vi "AI@ClassifyEditor__Parameter.vi"(1 "ParamterIn":string) -> (0 "ParamterOut":string)   [LabVIEW 2020]
uses:
  MainFrame/Global.vi
  <vilib>/vision/NI_Vision_Development_Module.lvlib
panel:
  out "Image":T1(plugin-control)
  in  "Preview":bool
  in  "SubDir":string(combo)
  in  "Capture":string(combo)
  in  "Confirm":bool
  # "AI@ClassifyEditor $Capture(\\$Directory)"
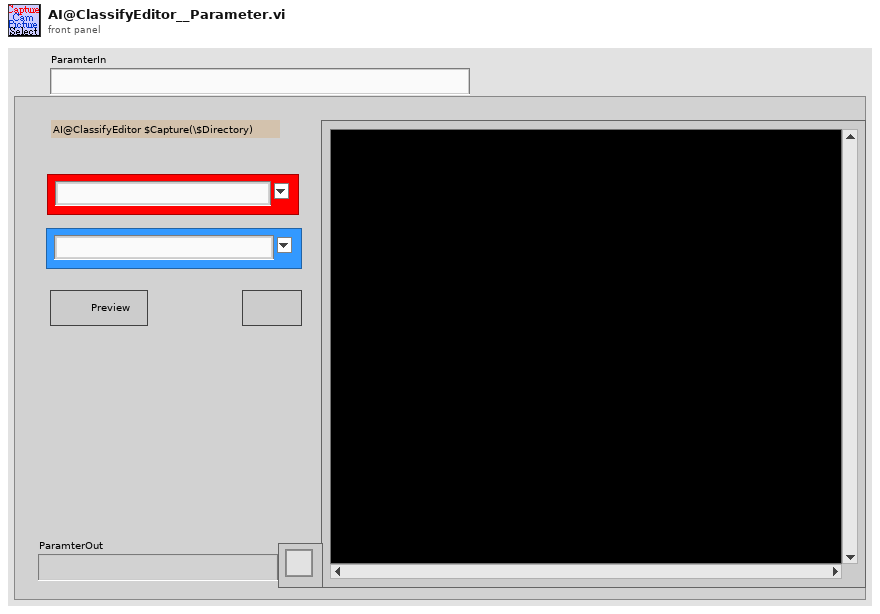
[diagram p1: front panel]
types:
  T1 = typedef "IMAQ Image.ctl" = refnum<image>
  T2 = cluster{"Browser Size":cluster{"X":i32, "Y":i32}, "Images per Line":i32, "Background Color":u32, "Frame Size":i32, "Frame Style":u16}
  T3 = typedef "Image Type" = u32
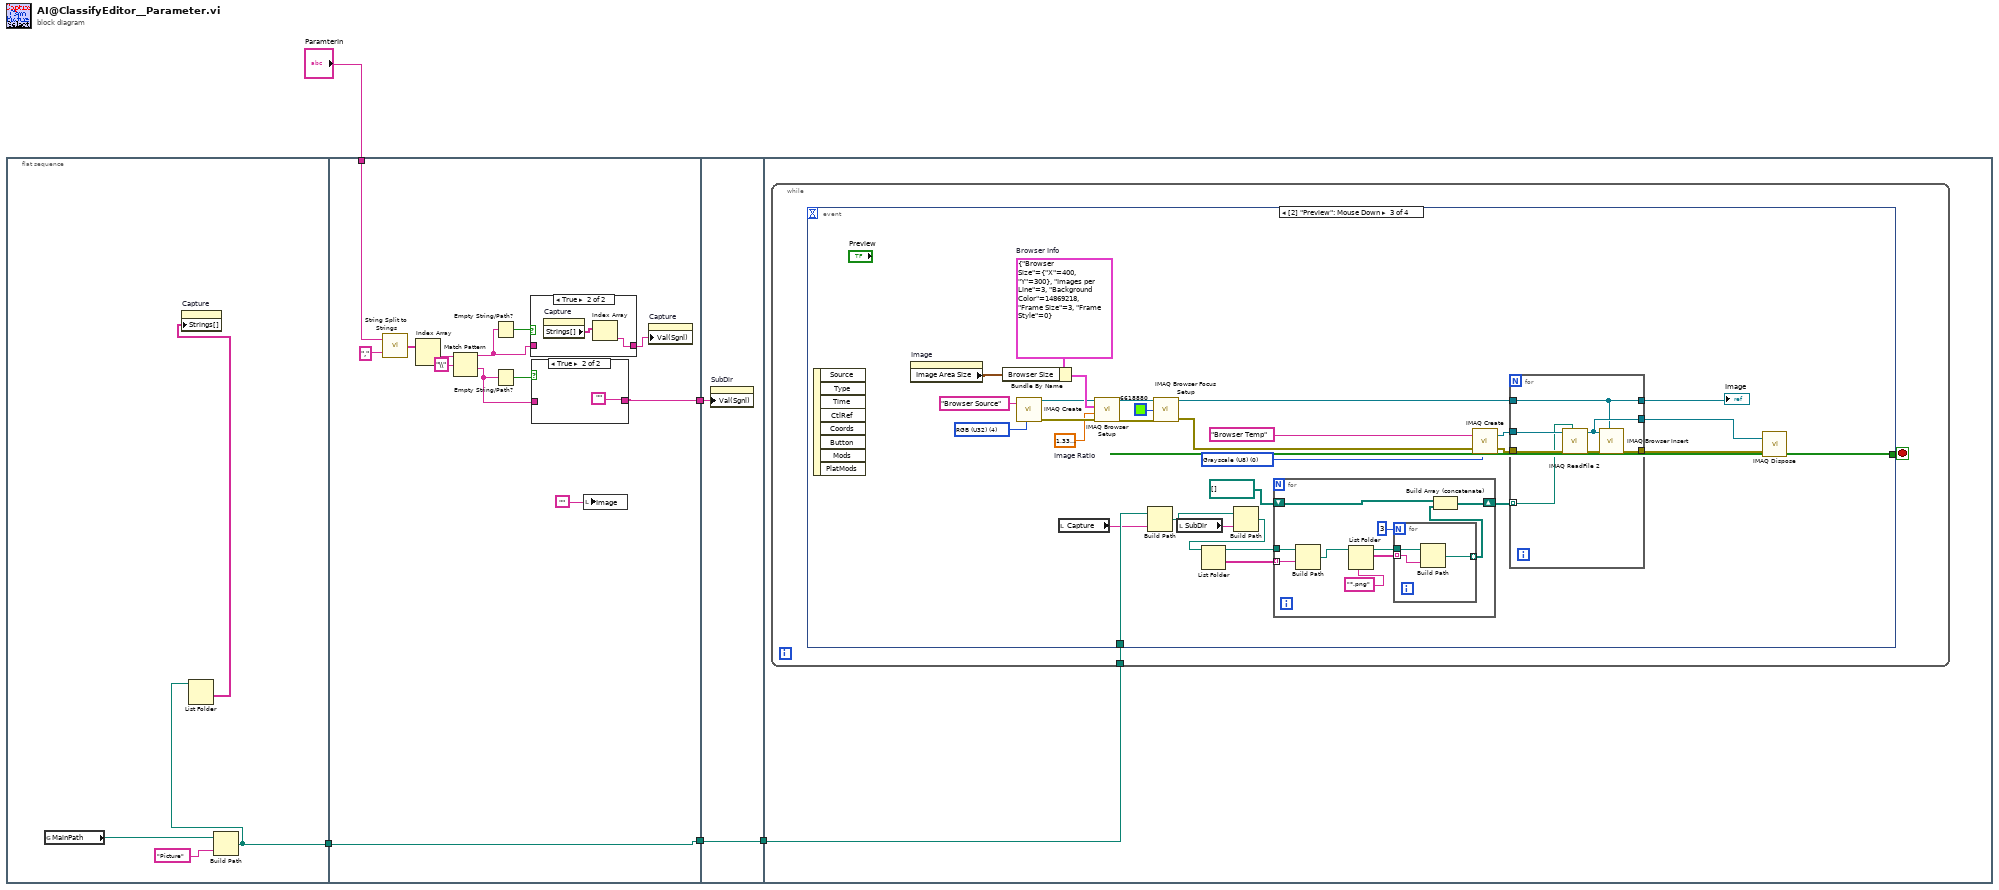
[diagram p0: block diagram]
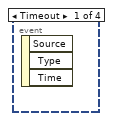
[diagram p4: hidden frame]
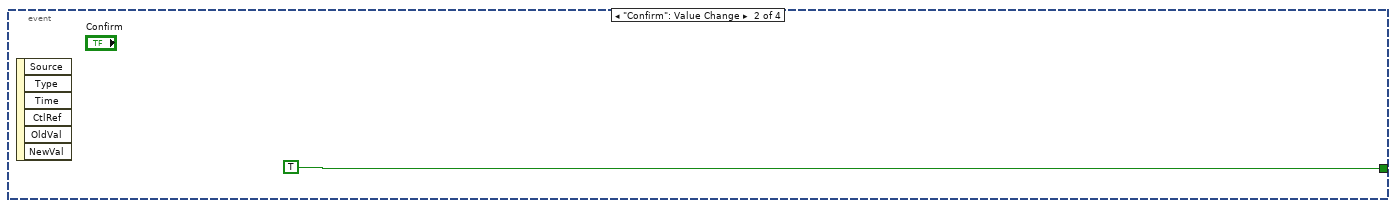
[diagram p5: hidden frame]
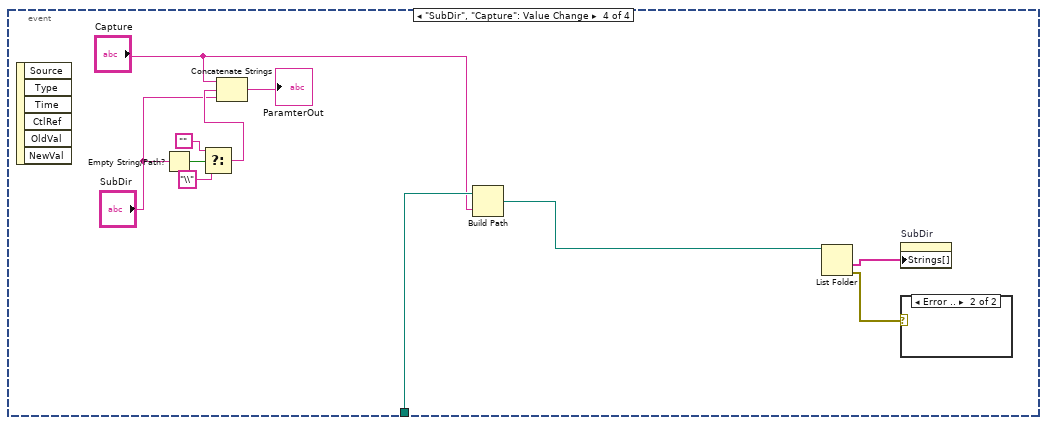
[diagram p6: hidden frame]
diagram:
  n1 = flat-sequence {
    tunnel: [w7] -> w2
    tunnel: "ParamterIn" -> [w20]
    tunnel: [w18] -> w3
    tunnel: w2 -> [w18]
    tunnel: [w17] -> w1
    tunnel: [w29] -> w4
    tunnel: w3 -> [w29]
    tunnel: w1 -> [w28]
    tunnel: w4 -> [w30]
    frame #0 {
      n2 = global read "Global.vi" "MainPath"() -> (w8:path)
      n3 = Build Path(base path=w8, name or relative path="Picture") -> (appended path=w7:path)
      n4 = List Folder(path=w7) -> (folder names=w6:string[])  [unwired: 3 in, 3 out]
      n5 = property on="Capture" class="CmbBox"("Strings[]"=w6) -> ()  [unwired: 2 in, 2 out]
    }
    frame #1 {
      n6 = call "String Split to Strings.vi"("search string/char (-)"=",", "String"=w20) -> ("Array"=w22:string[])
      n7 = Index Array(array=w22) -> (element #1=w14:string)  [unwired: 2 in, 1 out]
      n8 = Match Pattern(string=w14, regular expression="\\") -> (before substring=w12:string, after substring=w11:string)  [unwired: 1 in, 2 out]
      n9 = Empty String/Path?(string/path=w12) -> (empty?=w19:bool)
      n10 = Empty String/Path?(string/path=w11) -> (empty?=w15:bool)
      n11 = case shown="True" w19 {
        tunnel: w12 -> [w25 _]
        tunnel: [w25 w26] -> w16
        frame False {
        }
        frame True {
          n12 = property on="Capture" class="CmbBox"() -> ("Strings[]"=w27:string[])  [unwired: 2 in, 2 out]
          n13 = Index Array(array=w27) -> (element=w26:string)  [unwired: 1 in]
        }
      }
      n14 = case shown="True" w15 {
        tunnel: [w23 ""] -> w17
        tunnel: w11 -> [w23 _]
        frame False {
        }
        frame True {
        }
      }
      n15 = local write "Image"("") -> ()
      n16 = property on="Capture" class="CmbBox"("Val(Sgnl)"=w16) -> ()  [unwired: 2 in, 2 out]
    }
    frame #2 {
      n17 = property on="SubDir" class="CmbBox"("Val(Sgnl)"=w28) -> ()  [unwired: 2 in, 2 out]
    }
    frame #3 {
      n18 = while {
        tunnel: w30 -> [w31]
        stop <- w32 stop-if-true
        n19 = event shown="[2] \"Preview\": Mouse Down" {
          selector: _ -> [_ _ _ _]
          dyn-events: _ -> [_ _ _ _]
          timeout: _ -> [_ _ _ _]
          tunnel: [_ TRUE _ _] -> w32
          tunnel: w31 -> [_ _ w41 w91]
          event Timeout {
            n20 = event-data() -> ()  [unwired: 1 in, 3 out]
          }
          event "Confirm": Value Change {
            n21 = event-data() -> ()  [unwired: 1 in, 6 out]
          }
          event "Preview": Mouse Down {
            w43 = sgl 1.33  # Image Ratio
            w59 = T2 {"Browser Size"={"X"=400, "Y"=300}, "Images per Line"=3, "Background Color"=14869218, "Frame Size"=3, "Frame Style"=0}  # Browser Info
            w50 = T3 0 items=["Grayscale (U8)", "Grayscale (I16)", "Grayscale (SGL)", "Complex (CSG)", "RGB (U32)", "HSL (U32)", "RGB (U64)", "Grayscale (U16)"] ("Image Type")
            w48 = T3 4 items=["Grayscale (U8)", "Grayscale (I16)", "Grayscale (SGL)", "Complex (CSG)", "RGB (U32)", "HSL (U32)", "RGB (U64)", "Grayscale (U16)"] ("Image Type")
            n22 = event-data() -> ()  [unwired: 1 in, 8 out]
            n23 = property on="Image" class="ImageControl"() -> ("Image Area Size"=w60:cluster{"Width":u32, "Height":u32})  [unwired: 2 in, 2 out]
            n24 = Bundle By Name(cluster=w59, "Browser Size"=w60) -> (w61:T2)
            n25 = call "IMAQ Create"("Image Name"="Browser Source", "Image Type"=w48) -> ("New Image"=w46:T1, "error out"=w47:errorcluster)  [unwired: 3 in]
            n26 = local read "Capture"() -> (w40:string)
            n27 = call "IMAQ Browser Setup"("error in (no error)"=w47, "Image Ratio"=w43, "Browser Info"=w61, "Image In"=w46) -> ("error out"=w55:errorcluster, "Image Browser Out"=w54:T1)  [unwired: 2 out]
            n28 = Build Path(base path=w41, name or relative path=w40) -> (appended path=w39:path)
            n29 = call "IMAQ Browser Focus Setup"("error in (no error)"=w55, "Focus Color"=u32 6618880, "Image Browser In"=w54) -> ("error out"=w57:errorcluster, "Image Browser Out"=w56:T1)  [unwired: 1 in]
            n30 = local read "SubDir"() -> (w42:string)
            n31 = Build Path(base path=w39, name or relative path=w42) -> (appended path=w38:path)
            n32 = List Folder(path=w38) -> (path out=w37:path, folder names=w36:string[])  [unwired: 3 in, 2 out]
            n33 = for {
              tunnel: w37 -> [w65]
              tunnel: w36 -> [w64] mode=indexing
              shift-right: [w67] -> w34
              shift-left: path[] [] -> [w66]
              n34 = Build Path(base path=w65, name or relative path=w64) -> (appended path=w63:path)
              n35 = List Folder(path=w63, pattern="*.png") -> (path out=w70:path, filenames=w69:string[])  [unwired: 2 in, 2 out]
              n36 = for {
                N: 3 -> [_]
                tunnel: w70 -> [w75]
                tunnel: w69 -> [w74] mode=indexing
                tunnel: [w73] -> w68 mode=indexing
                n37 = Build Path(base path=w75, name or relative path=w74) -> (appended path=w73:path)
              }
              n38 = Build Array (concatenate)(w66, w68) -> (w67:path[])
            }
            n39 = call "IMAQ Create"("Image Name"="Browser Temp", "Image Type"=w50, "error in (no error)"=w57) -> ("New Image"=w52:T1, "error out"=w44:errorcluster)  [unwired: 2 in]
            n40 = for {
              tunnel: w56 -> [w77]
              tunnel: w44 -> [w81]
              tunnel: [w80] -> w45
              tunnel: [w77] -> w62
              tunnel: w52 -> [w79]
              tunnel: [w78] -> w53
              tunnel: w34 -> [w76] mode=indexing
              n41 = call "IMAQ ReadFile 2"("File Path"=w76, "error in (no error)"=w81, "Image"=w79) -> ("error out"=w82:errorcluster, "Image Out"=w78:T1)  [unwired: 4 in, 3 out]
              n42 = call "IMAQ Browser Insert"("Image Browser In"=w77, "error in (no error)"=w82, "Image to Add"=w78) -> ("error out"=w80:errorcluster)  [unwired: 4 in, 4 out]
            }
            "Image" <- w62
            n43 = call "IMAQ Dispose"("Image"=w53, "error in (no error)"=w45) -> ()  [unwired: 4 in, 1 out]
          }
          event "SubDir", "Capture": Value Change {
            n44 = event-data() -> ()  [unwired: 1 in, 6 out]
            n45 = Empty String/Path?(string/path="SubDir") -> (empty?=w87:bool)
            n46 = Select(t="", s=w87, f="\\" ("string")) -> (s? t:f=w84:string)
            n47 = Concatenate Strings("Capture", w84, "SubDir") -> (→"ParamterOut":string)
            n48 = Build Path(base path=w91, name or relative path="Capture") -> (appended path=w90:path)
            n49 = List Folder(path=w90) -> (folder names=w89:string[], error out=w92:errorcluster)  [unwired: 3 in, 2 out]
            n50 = property on="SubDir" class="CmbBox"("Strings[]"=w89) -> ()  [unwired: 2 in, 2 out]
            n51 = case shown="Error .." w92 {
              frame No Error {
              }
              frame Error {
              }
            }
          }
        }
      }
    }
  }
